vi "StartFastChannelStreaming.vi"(4 "dt":dbl, 5 "t0":dbl, 6 "group name in (Untitled)":string="Untitled", 7 "channel name(s) in (Untitled)":string, 8 "error in (no error)":errorcluster, 9 "Scaling coefficients":dbl[](array[numeric]), 10 "Data":i16[](array[numeric]), 11 "tdms file":refnum<k34>) -> (0 "error out":errorcluster, 3 "tdms file out":refnum<k34>)   [LabVIEW 2015]
uses:
  <vilib>/Utility/tdmsutil.llb/TDMS Create Scaling Information (Linear).vi
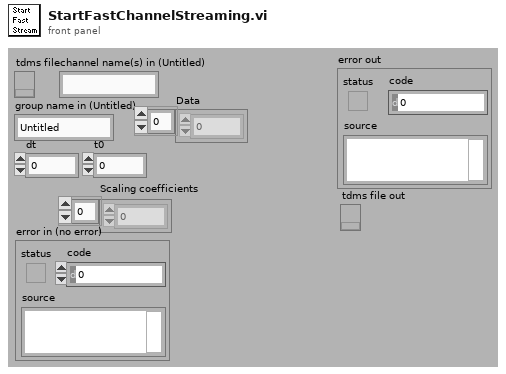
[diagram p1: front panel]
types:
  T1 = cluster{"slope":dbl, "y intercept":dbl, "input source":i32}
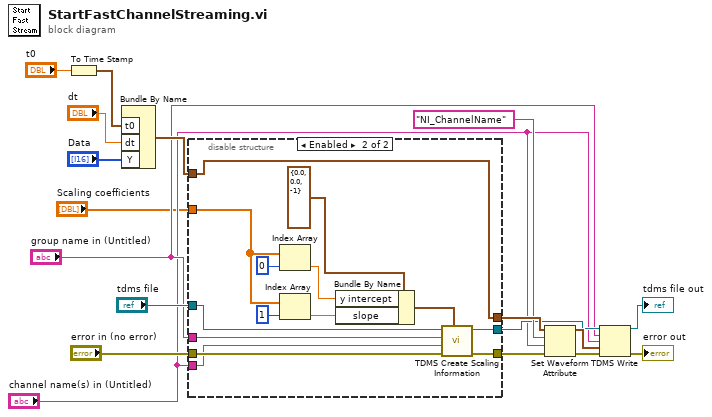
[diagram p0: block diagram]
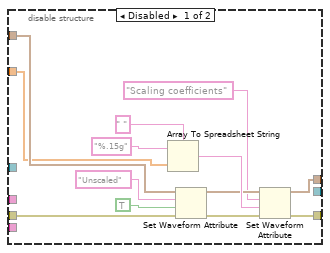
[diagram p2: hidden frame]
diagram:
  n1 = To Time Stamp(1:"t0") -> (0:w18:timestamp)
  n2 = Bundle By Name("t0"=w18, "dt"="dt", "Y"="Data") -> (w16:waveform(i16))  [unwired: 1 out]
  n3 = disable-structure shown="Enabled" {
    disable-tunnel: w16 -> [w25 w42]
    disable-tunnel: [w22 w45] -> w11
    disable-tunnel: [w21 w42] -> w8
    disable-tunnel: "error in (no error)" -> [w19 w44]
    disable-tunnel: "tdms file" -> [_ w43]
    disable-tunnel: [_ w41] -> w4
    disable-tunnel: "group name in (Untitled)" -> [_ w40]
    disable-tunnel: "channel name(s) in (Untitled)" -> [_ w39]
    disable-tunnel: "Scaling coefficients" -> [w20 w33]
    frame Disabled {
      n4 = Array To Spreadsheet String(delimiter (Tab)=" ", array=w20, 3:"%.15g" ("format string")) -> (spreadsheet string=w29:string)
      n5 = Set Waveform Attribute(4:w19, 5:TRUE, 6:"Unscaled" ("name"), 7:w25) -> (0:w26:errorcluster, 3:w24:waveform(i16))  [unwired: 1 out]
      n6 = Set Waveform Attribute(4:w26, 5:w29, 6:"Scaling coefficients", 7:w24) -> (0:w22:errorcluster, 3:w21:waveform(i16))  [unwired: 1 out]
    }
    frame Enabled {
      n7 = Index Array(array=w33, index=0) -> (element=w35:dbl)
      n8 = Index Array(array=w33, index=1) -> (element=w34:dbl)
      n9 = Bundle By Name(cluster=T1 {"slope"=0.0, "y intercept"=0.0, "input source"=-1} ("linear scale"), "y intercept"=w35, "slope"=w34) -> (w38:T1)
      n10 = call-poly <vilib>:"TDMS Create Scaling Information.vi"("linear scale"=w38, "error in (no error)"=w44, "channel name"=w39, "group name"=w40, "tdms file"=w43) -> ("error out"=w45:errorcluster, "tdms file out"=w41:refnum<k34>)  [unwired: 2 in, 3 out]
    }
  }
  n11 = Set Waveform Attribute(4:w11, 5:"channel name(s) in (Untitled)", 6:"NI_ChannelName", 7:w8) -> (0:w10:errorcluster, 3:w9:waveform(i16))  [unwired: 1 out]
  n12 = TDMS Write(0:w4, 5:"group name in (Untitled)", 7:"channel name(s) in (Untitled)", 9:w9, 11:w10) -> (4:→"tdms file out":refnum<k34>, 15:→"error out":errorcluster)  [unwired: 1 in, 2 out]
